vi "DHE_DACS_Alias_parse_request.vi"(10 "cmd in":string) -> (0 "number of points":i32, 1 "mult. aliases?":bool, 2 "cmds out":string[](array[string]), 3 "alias names":string[](array[string]))   [LabVIEW 2016]
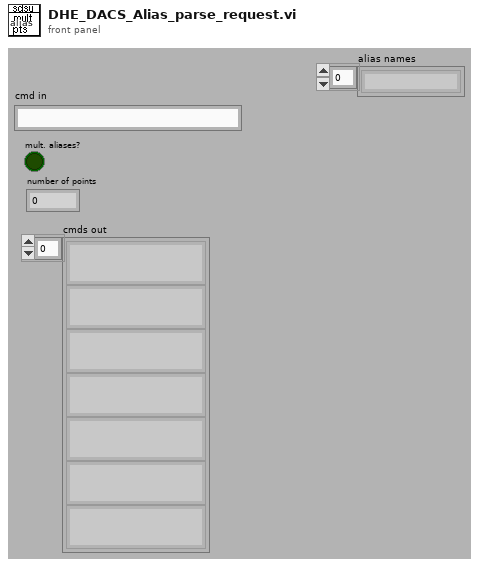
[diagram p1: front panel]
types:
  T1 = enum16{"read from file", "find", "get", "add", "delete", "clear "}
  T2 = typedef "DHE_alias.ctl" = cluster{"alias":string, "varout set":string, "varout get":string}
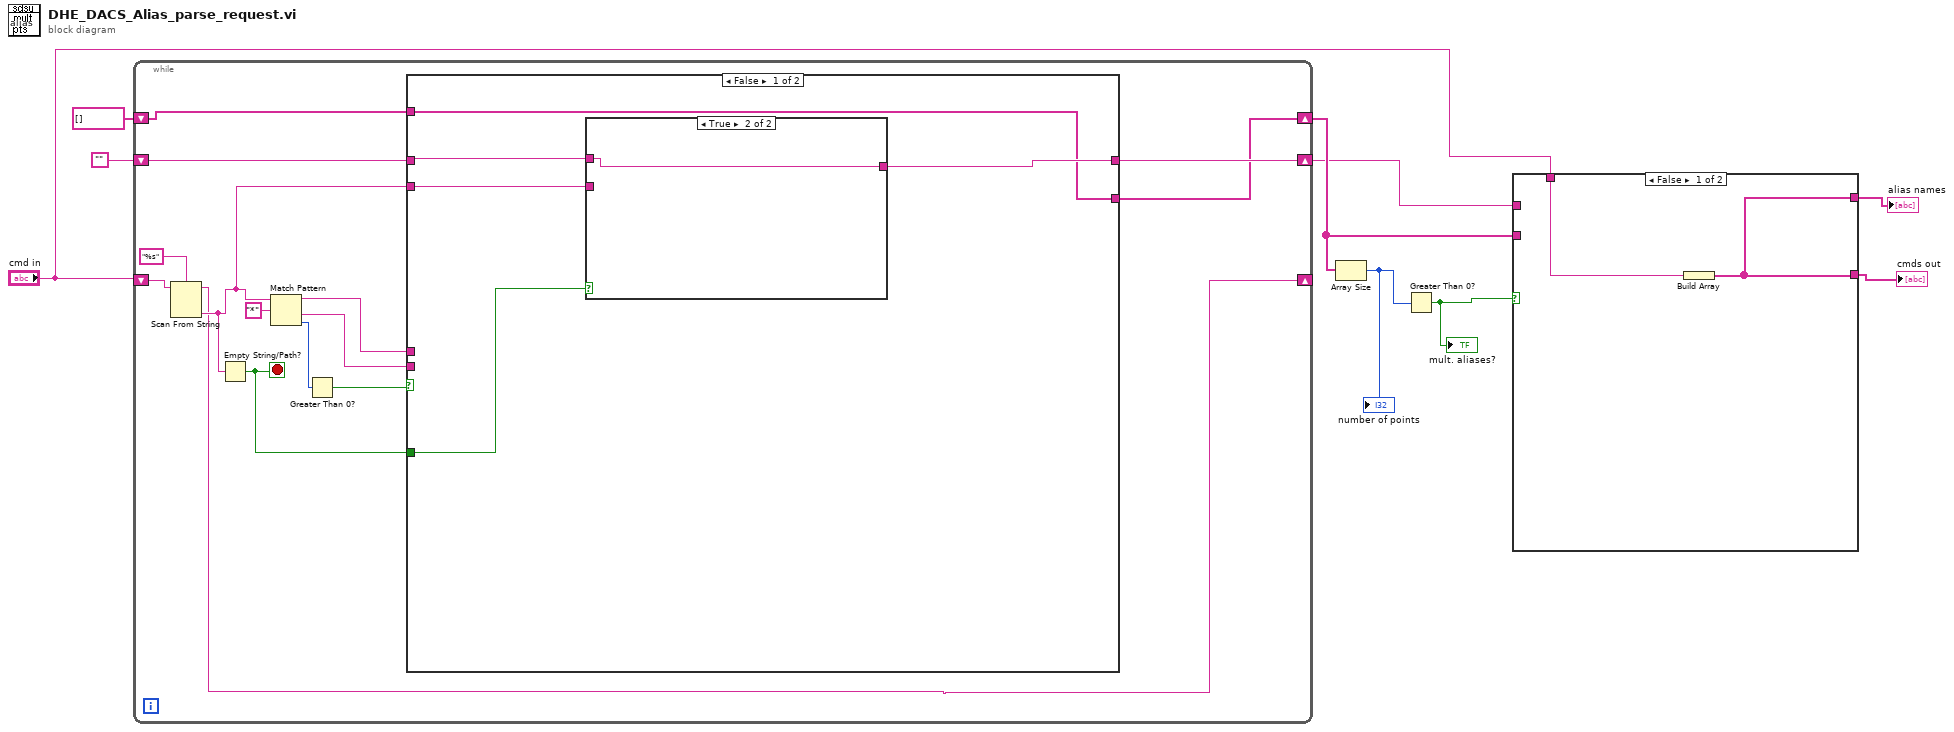
[diagram p0: block diagram]
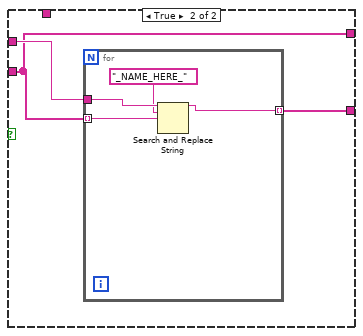
[diagram p2: hidden frame]
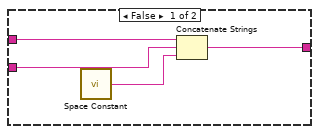
[diagram p3: hidden frame]
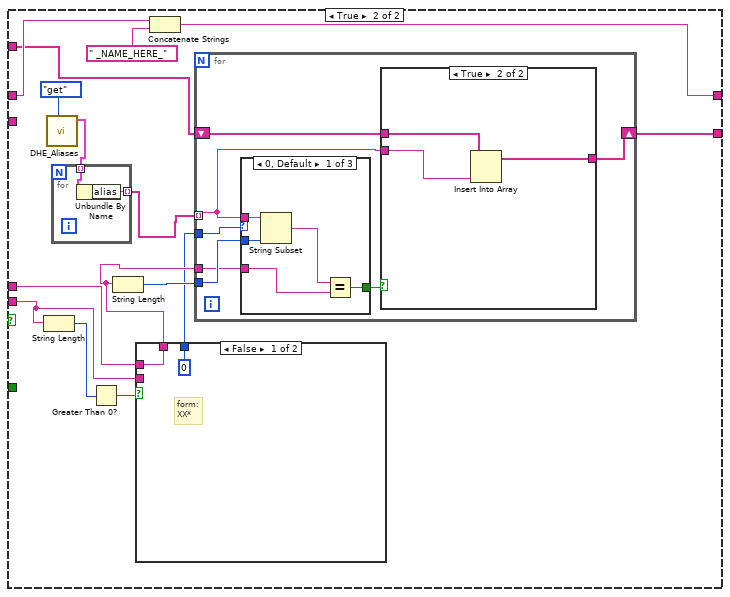
[diagram p4: hidden frame]
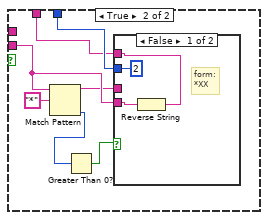
[diagram p5: hidden frame]
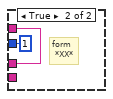
[diagram p6: hidden frame]
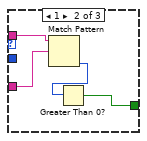
[diagram p7: hidden frame]
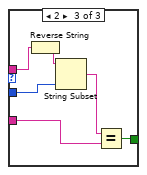
[diagram p8: hidden frame]
diagram:
  n1 = while {
    shift-right: [w12] -> _
    shift-left: "cmd in" -> [w18]
    shift-right: [w15] -> w2
    shift-left: "" -> [w16]
    shift-right: [w11] -> w5
    shift-left: string[] [] -> [w10]
    stop <- w13 stop-if-true
    n2 = Scan From String(format string="%s", input string=w18) -> (remaining string=w12:string, output 1=w14:string)  [unwired: 3 in, 2 out]
    n3 = Empty String/Path?(string/path=w14) -> (empty?=w13:bool)
    n4 = Match Pattern(string=w14, regular expression="*") -> (before substring=w20:string, after substring=w19:string, offset past match=w22:i32)  [unwired: 2 out]
    n5 = Greater Than 0?(x=w22) -> (x > 0?=w21:bool)
    n6 = case shown="False" w21 {
      tunnel: w20 -> [_ w43]
      tunnel: [w24 w47] -> w11
      tunnel: w19 -> [_ w44]
      tunnel: w16 -> [w28 w37]
      tunnel: w14 -> [w27 _]
      tunnel: [w26 w35] -> w15
      tunnel: w13 -> [w25 _]
      tunnel: w10 -> [w24 w34]
      frame False {
        n7 = case shown="True" w25 {
          tunnel: w28 -> [w32 w33]
          tunnel: w27 -> [w31 _]
          tunnel: [w29 w33] -> w26
          frame False {
            n8 = call <vilib>:"Space Constant.vi"() -> ("String"=w30:string)
            n9 = Concatenate Strings(w32, w31, w30) -> (w29:string)
          }
          frame True {
          }
        }
      }
      frame True {
        n10 = String Length(string=w44) -> (length=w46:i32)
        n11 = call "DHE_Aliases.vi"("action"=T1."get") -> ("aliases"=w39:T2[])  [unwired: 7 in, 3 out]
        n12 = for {
          tunnel: w39 -> [w50] mode=indexing
          tunnel: [w49] -> w38 mode=indexing
          n13 = Unbundle By Name(w50) -> ("alias"=w49:string)
        }
        n14 = Greater Than 0?(x=w46) -> (x > 0?=w45:bool)
        n15 = case shown="False" w45 {
          tunnel: w44 -> [_ w55]
          tunnel: w43 -> [w52 _]
          tunnel: [w52 w53] -> w42
          tunnel: [0 w56] -> w41
          frame False {
            # "form:\nXX*"
          }
          frame True {
            n16 = Match Pattern(string=w55, regular expression="*") -> (before substring=w54:string, offset past match=w58:i32)  [unwired: 3 out]
            n17 = Greater Than 0?(x=w58) -> (x > 0?=w57:bool)
            n18 = case shown="False" w57 {
              tunnel: [2 1] -> w56
              tunnel: w55 -> [w61 _]
              tunnel: w54 -> [_ w63]
              tunnel: [w60 w63] -> w53
              frame False {
                # "form:\n*XX"
                n19 = Reverse String(1:w61) -> (0:w60:string)
              }
              frame True {
                # "form\n *XX*"
              }
            }
          }
        }
        n20 = String Length(string=w42) -> (length=w48:i32)
        n21 = Concatenate Strings(w37, " _NAME_HERE_" ("string")) -> (w35:string)
        n22 = for {
          tunnel: w42 -> [w70]
          tunnel: w38 -> [w68] mode=indexing
          tunnel: w48 -> [w71]
          shift-right: [w67] -> w47
          shift-left: w34 -> [w66]
          tunnel: w41 -> [w65]
          n23 = case shown="0, Default" w65 {
            tunnel: w71 -> [w76 _ w84]
            tunnel: w70 -> [w75 w79 w82]
            tunnel: [w74 w77 w81] -> w69
            tunnel: w68 -> [w72 w80 w86]
            frame 0, Default {
              n24 = String Subset(string=w72, length (rest)=w76) -> (substring=w73:string)  [unwired: 1 out]
              n25 = Equal?(x=w73, y=w75) -> (x = y?=w74:bool)
            }
            frame 1 {
              n26 = Match Pattern(string=w80, regular expression=w79) -> (offset past match=w78:i32)  [unwired: 4 out]
              n27 = Greater Than 0?(x=w78) -> (x > 0?=w77:bool)
            }
            frame 2 {
              n28 = Reverse String(1:w86) -> (0:w85:string)
              n29 = String Subset(string=w85, length (rest)=w84) -> (substring=w83:string)  [unwired: 1 out]
              n30 = Equal?(x=w83, y=w82) -> (x = y?=w81:bool)
            }
          }
          n31 = case shown="True" w69 {
            tunnel: w68 -> [_ w90]
            tunnel: [w87 w89] -> w67
            tunnel: w66 -> [w87 w88]
            frame False {
            }
            frame True {
              n32 = Insert Into Array(array=w88, new element=w90) -> (w89:string[])  [unwired: 1 in]
            }
          }
        }
      }
    }
  }
  n33 = Array Size(array=w5) -> (size(s)=w6:i32)
  "number of points" <- w6
  n34 = Greater Than 0?(x=w6) -> (x > 0?=w7:bool)
  "mult. aliases?" <- w7
  n35 = case shown="False" w7 {
    tunnel: "cmd in" -> [w92 _]
    tunnel: w5 -> [_ w93]
    tunnel: [w91 w95] -> w8
    tunnel: w2 -> [_ w94]
    tunnel: [w91 w93] -> w1
    frame False {
      n36 = Build Array(w92) -> (w91:string[])
    }
    frame True {
      n37 = for {
        tunnel: w93 -> [w97] mode=indexing
        tunnel: w94 -> [w99]
        tunnel: [w96] -> w95 mode=indexing
        n38 = Search and Replace String(input string=w99, search string="_NAME_HERE_" ("string"), replace string=w97) -> (result string=w96:string)  [unwired: 5 in, 3 out]
      }
    }
  }
  "cmds out" <- w8
  "alias names" <- w1
